vi "Get Location.vi"(11 "Class":refnum<class "Pinwheel.lvclass">) -> (0 "Clan":T1, 1 "Post":T1, 2 "Ring":T3, 3 "Class":refnum<class "Pinwheel.lvclass">, 4 "Diagonal":bool, 5 "OD":T1, 6 "Role":T2, 7 "Jump":bool, 8 "Move Anyway":bool, 10 "Chute":bool)   [LabVIEW 2020, in "Pinwheel.lvclass"]
uses:
  Pinwheel.lvclass
  Ring Enum.ctl
  Type Defs/Direction Enum.ctl
  Role Enum.ctl
  Pinwheel.lvclass/Pinwheel.ctl
  Type Defs/SB Type Defs.lvlib
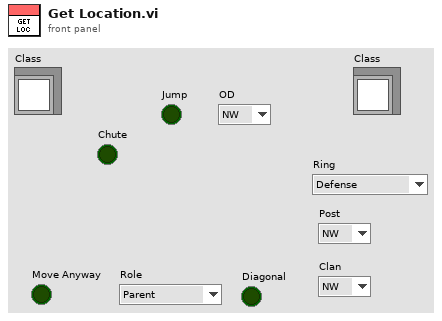
[diagram p1: front panel]
types:
  T1 = typedef "SB Type Defs.lvlib/Direction Enum.ctl" = enum16{"NW", "N", "NE", "E", "SE", "S", "SW", "W"}
  T2 = typedef "Pinwheel.lvclass/Role Enum.ctl" = enum16{"Parent", "Move", "Child"}
  T3 = typedef "Pinwheel.lvclass/Ring Enum.ctl" = enum16{"Defense", "Fill", "Outer", "Inner"}
  T4 = typedef "Pinwheel.lvclass/DVR Cluster.ctl" = cluster{"N":i32, "E":i32, "S":i32, "W":i32, "OD":T1, "NR":i32, "ER":i32, "SR":i32, "WR":i32, "NE":i32, "EE":i32, "SE":i32, "WE":i32, "Team":i32}
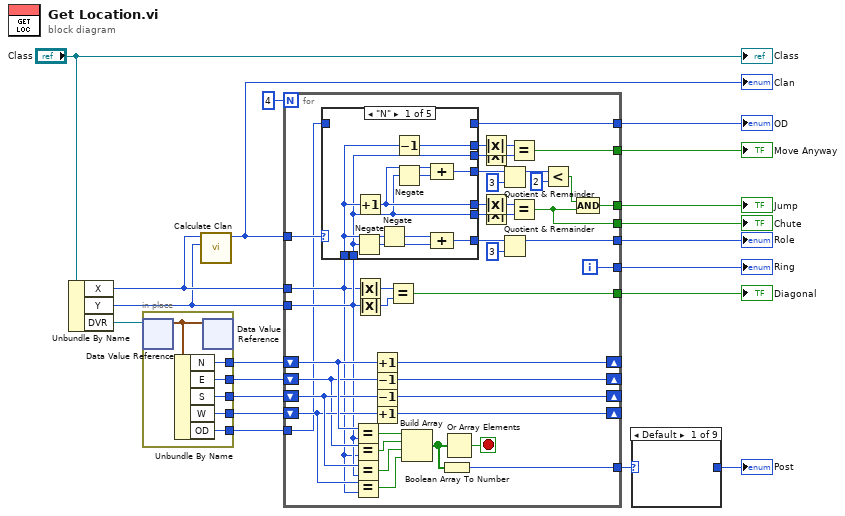
[diagram p0: block diagram]
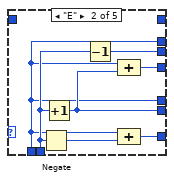
[diagram p2: hidden frame]
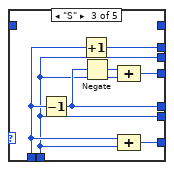
[diagram p3: hidden frame]
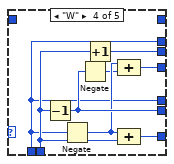
[diagram p4: hidden frame]
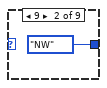
[diagram p6: hidden frame]
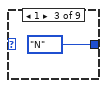
[diagram p7: hidden frame]
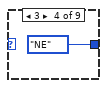
[diagram p8: hidden frame]
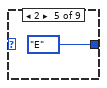
[diagram p9: hidden frame]
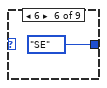
[diagram p10: hidden frame]
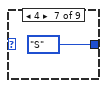
[diagram p11: hidden frame]
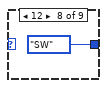
[diagram p12: hidden frame]
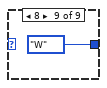
[diagram p13: hidden frame]
diagram:
  n1 = Unbundle By Name("Class") -> ("X"=w4:i32, "Y"=w3:i32, "DVR"=w20:refnum<data-value>)
  n2 = in-place {
    in-place-border: [w25] -> w6
    in-place-border: [w24] -> w8
    in-place-border: [w23] -> w5
    in-place-border: [w22] -> w7
    in-place-border: [w21] -> w13
    n3 = in-place-dvr #1(w20) -> (w26:T4)  [unwired: 1 out]
    n4 = Unbundle By Name(w26) -> ("N"=w25:i32, "E"=w24:i32, "S"=w23:i32, "W"=w22:i32, "OD"=w21:T1)
    n5 = in-place-dvr #1(w26) -> ()  [unwired: 2 out]
  }
  n6 = call "Calculate Clan.vi"("Y"=w3, "X"=w4) -> ("Clan"=w2:T1)  [unwired: 9 in]
  "Clan" <- w2
  n7 = for {
    N: 4 -> [_]
    tunnel: w3 -> [w59]
    tunnel: w4 -> [w58]
    tunnel: [w56] -> w11
    shift-right: [w68] -> _
    shift-left: w6 -> [w69]
    shift-right: [w62] -> _
    shift-left: w8 -> [w63]
    shift-right: [w66] -> _
    shift-left: w5 -> [w67]
    shift-right: [w64] -> _
    shift-left: w7 -> [w65]
    tunnel: [w60] -> w18
    tunnel: [w57] -> w17
    tunnel: [w55] -> w16
    tunnel: w2 -> [w54]
    tunnel: [w53] -> w15
    tunnel: [w52] -> w14
    tunnel: w13 -> [w51]
    tunnel: [w50] -> w12
    tunnel: [w49] -> w9
    i -> [w56]
    stop <- w61 stop-if-true
    n8 = case shown="\"N\"" w54 {
      tunnel: w58 -> [w72 w80 w90 w94 _]
      tunnel: w59 -> [w71 w82 w87 w98 _]
      tunnel: [w78 w85 w92 w100 _] -> w48
      tunnel: [_ _ _ _ w101] -> w53
      tunnel: [w71 w81 w87 w97 _] -> w44
      tunnel: [w73 w80 w89 w94 _] -> w43
      tunnel: w51 -> [_ _ _ _ w101]
      tunnel: [w70 w80 w86 w94 _] -> w38
      tunnel: [w71 w79 w87 w93 _] -> w37
      tunnel: [w76 w84 w91 w99 _] -> w35
      frame "N" {
        n9 = Negate(x=w71) -> (-x=w75:i32)
        n10 = Increment(x=w72) -> (x+1=w73:i32)
        n11 = Negate(x=w72) -> (-x=w77:i32)
        n12 = Decrement(x=w72) -> (x-1=w70:i32)
        n13 = Negate(x=w71) -> (-x=w74:i32)
        n14 = Compound Arithmetic op=ADD(w73, w74) -> (w76:i32)
        n15 = Compound Arithmetic op=ADD(w77, w75) -> (w78:i32)
      }
      frame "E" {
        n16 = Negate(x=w82) -> (-x=w83:i32)
        n17 = Increment(x=w82) -> (x+1=w81:i32)
        n18 = Decrement(x=w82) -> (x-1=w79:i32)
        n19 = Compound Arithmetic op=ADD(w80, w81) -> (w84:i32)
        n20 = Compound Arithmetic op=ADD(w80, w83) -> (w85:i32)
      }
      frame "S" {
        n21 = Decrement(x=w90) -> (x-1=w89:i32)
        n22 = Increment(x=w90) -> (x+1=w86:i32)
        n23 = Negate(x=w89) -> (-x=w88:i32)
        n24 = Compound Arithmetic op=ADD(w88, w87) -> (w91:i32)
        n25 = Compound Arithmetic op=ADD(w90, w87) -> (w92:i32)
      }
      frame "W" {
        n26 = Decrement(x=w98) -> (x-1=w97:i32)
        n27 = Negate(x=w94) -> (-x=w96:i32)
        n28 = Negate(x=w97) -> (-x=w95:i32)
        n29 = Increment(x=w98) -> (x+1=w93:i32)
        n30 = Compound Arithmetic op=ADD(w96, w95) -> (w99:i32)
        n31 = Compound Arithmetic op=ADD(w96, w98) -> (w100:i32)
      }
      frame Default {
      }
    }
    n32 = Equal?(x=w69, y=w59) -> (x = y?=w31:bool)
    n33 = Equal?(x=w63, y=w58) -> (x = y?=w30:bool)
    n34 = Equal?(x=w67, y=w59) -> (x = y?=w29:bool)
    n35 = Equal?(x=w65, y=w58) -> (x = y?=w28:bool)
    n36 = Absolute Value(x=w58) -> (abs(x)=w45:i32)
    n37 = Absolute Value(x=w59) -> (abs(x)=w46:i32)
    n38 = Increment(x=w69) -> (x+1=w68:i32)
    n39 = Decrement(x=w63) -> (x-1=w62:i32)
    n40 = Decrement(x=w67) -> (x-1=w66:i32)
    n41 = Increment(x=w65) -> (x+1=w64:i32)
    n42 = Equal?(x=w45, y=w46) -> (x = y?=w57:bool)
    n43 = Build Array(w31, w30, w29, w28) -> (w27:bool[])
    n44 = Boolean Array To Number(Boolean array=w27) -> (number=w60:u32)
    n45 = Or Array Elements(Boolean array=w27) -> (logical OR=w61:bool)
    n46 = Absolute Value(x=w38) -> (abs(x)=w39:i32)
    n47 = Absolute Value(x=w37) -> (abs(x)=w40:i32)
    n48 = Absolute Value(x=w43) -> (abs(x)=w42:i32)
    n49 = Absolute Value(x=w44) -> (abs(x)=w41:i32)
    n50 = Quotient & Remainder(x=w35, y=3) -> (x-y*floor(x/y)=w34:i32)  [unwired: 1 out]
    n51 = Quotient & Remainder(x=w48, y=3) -> (x-y*floor(x/y)=w55:i32)  [unwired: 1 out]
    n52 = Equal?(x=w39, y=w40) -> (x = y?=w50:bool)
    n53 = Equal?(x=w42, y=w41) -> (x = y?=w49:bool)
    n54 = Less?(x=w34, y=2) -> (x < y?=w33:bool)
    n55 = Compound Arithmetic op=AND(w33, w49) -> (w52:bool)
  }
  "Ring" <- w11
  "Diagonal" <- w17
  "Role" <- w16
  "OD" <- w15
  "Jump" <- w14
  "Move Anyway" <- w12
  "Chute" <- w9
  n56 = case shown="Default" w18 {
    tunnel: [_ Direction_Enum."NW" ("Post") Direction_Enum."N" ("Post") Direction_Enum."NE" ("Post") Direction_Enum."E" ("Post") Direction_Enum."SE" ("Post") Direction_Enum."S" ("Post") Direction_Enum."SW" ("Post") Direction_Enum."W" ("Post")] -> w10
    frame Default {
    }
    frame 9 {
    }
    frame 1 {
    }
    frame 3 {
    }
    frame 2 {
    }
    frame 6 {
    }
    frame 4 {
    }
    frame 12 {
    }
    frame 8 {
    }
  }
  "Post" <- w10
  "Class" <- "Class"
